vi "Open visa first call.vi"(6 "Parity":u16(ring)=2 items=["None", "Odd", "Even", "Mark", "Space"], 8 "error in (no error)":errorcluster, 9 "error":bool, 10 "Com port":u8, 11 "VISA Refnum in":refnum<visa-resource-name>) -> (0 "error out":errorcluster, 3 "VISA Refnum out":refnum<visa-resource-name>)   [LabVIEW 2019]
panel:
  out "String":string
  out "find list":string[](array[string])
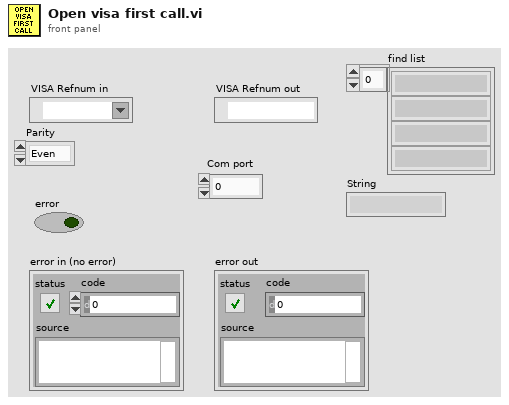
[diagram p1: front panel]
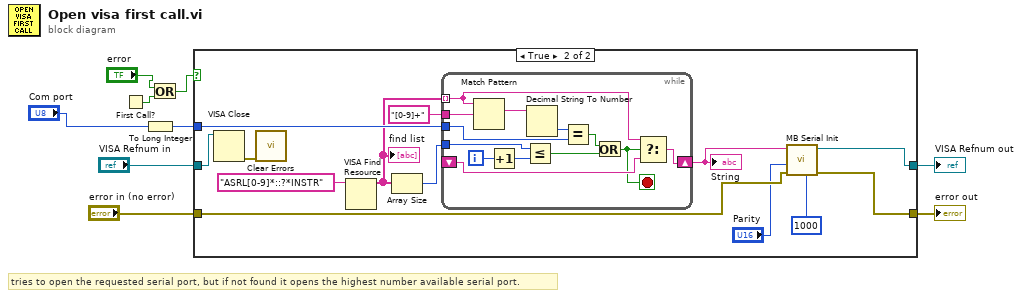
[diagram p0: block diagram]
diagram:
  # "tries to open the requested serial port, but if not found it opens the highest number available serial port."
  n1 = First Call?() -> (First Call?: T/F=w3:bool)
  n2 = To Long Integer(number="Com port") -> (32bit integer=w5:i32)
  n3 = Or(x="error", y=w3) -> (x .or. y?=w1:bool)
  n4 = case shown="True" w1 {
    tunnel: [w10 w16] -> w6
    tunnel: [w11 w13] -> w7
    tunnel: "error in (no error)" -> [w11 w14]
    tunnel: "VISA Refnum in" -> [w10 w22]
    tunnel: w5 -> [_ w20]
    frame False {
    }
    frame True {
      n5 = VISA Close(VISA resource name=w22) -> (error out=w21:errorcluster)  [unwired: 1 in]
      n6 = call <vilib>:"Clear Errors.vi"("error in (no error)"=w21) -> ()  [unwired: 5 in, 2 out]
      n7 = VISA Find Resource(11:"ASRL[0-9]*::?*INSTR" ("expression (\"?*\")")) -> (3:w19:string[])  [unwired: 2 in, 2 out]
      "find list" <- w19
      n8 = Array Size(array=w19) -> (size(s)=w18:i32)
      n9 = while {
        tunnel: w19 -> [w34] mode=indexing
        tunnel: w20 -> [w37]
        shift-right: [w35] -> w17
        shift-left: _ -> [w36]
        tunnel: "[0-9]+" ("regular expression") -> [w33]
        tunnel: w18 -> [w29]
        i -> [w30]
        stop <- w25 stop-if-true
        n10 = Match Pattern(string=w34, regular expression=w33) -> (match substring=w32:string)  [unwired: 1 in, 3 out]
        n11 = Increment(x=w30) -> (x+1=w26:i32)
        n12 = Less Or Equal?(x=w29, y=w26) -> (x <= y?=w27:bool)
        n13 = Decimal String To Number(string=w32) -> (number=w31:i32)  [unwired: 2 in, 1 out]
        n14 = Equal?(x=w31, y=w37) -> (x = y?=w28:bool)
        n15 = Or(x=w28, y=w27) -> (x .or. y?=w25:bool)
        n16 = Select(t=w34, s=w25, f=w36) -> (s? t:f=w35:string)
      }
      "String" <- w17
      n17 = call "MB Serial Init.vi"("Timeout"=u32 1000 ("General Settings:Timeout Value"), "error in (no error)"=w14, "Parity"="Parity", "VISA resource name"=w17) -> ("error out"=w13:errorcluster, "VISA resource name out"=w16:refnum<visa-resource-name>)  [unwired: 6 in]
    }
  }
  "error out" <- w7
  "VISA Refnum out" <- w6
